vi "PathfinderUtil_ToTrajectoryStates.vi"(11 "Pathfinder Path":T1[](array[typedef])) -> (3 "TrajectoryStates":T2[](array[typedef]) {"POSE"."ROTATION"."SIN" format="%13.4f"; "POSE"."ROTATION"."COS" format="%13.4f"; "POSE"."ROTATION"."VALUE" format="%13.4f"; "POSE"."TRANSLATION"."Y" format="%14.3f"; "POSE"."TRANSLATION"."X" format="%14.3f"})   [LabVIEW 2019, in "Trajectory_Library.lvlib"]
doc: "Convert an array of Pathfinder created Path states to an array of Trajectory States. Inches are converted to Meters. Angles are converted to headings (+/- PI). This routine only does a portion of the work needed to convert a Pathfinder Path to a complete Trajectory. (See PathfinderUtil_ToTrajectory for a complete routine.)\n\nParameters:\n - Pathfinder Path - Array of pathfinder created states\n\nReturns:\n - Trajectory States - Array of Trajectory states."
uses:
  Trajectory_Library.lvlib
  TRAJ_STATE.ctl
  POSE2D.ctl
  TRANSLATION2D.ctl
  ROTATION2D.ctl
  Pathfinder-Lib/VIs/Segment.ctl
  Rotation_CreateAngle.vi
  Translation_Create.vi
  Pathfinder-Lib/Pathfinder.lvlib
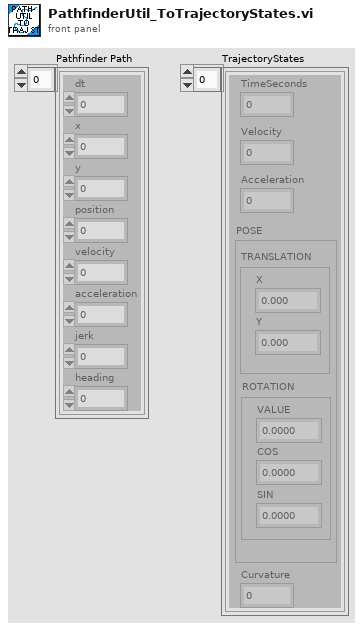
[diagram p1: front panel]
types:
  T1 = typedef "Pathfinder.lvlib/Segment.ctl" = cluster{"dt":dbl, "x":dbl, "y":dbl, "position":dbl, "velocity":dbl, "acceleration":dbl, "jerk":dbl, "heading":dbl}
  T2 = typedef "Trajectory_Library.lvlib/TRAJ_STATE.ctl" = cluster{"TimeSeconds":dbl, "Velocity":dbl, "Acceleration":dbl, "POSE":T3, "Curvature":dbl}
  T3 = typedef "Trajectory_Library.lvlib/POSE2D.ctl" = cluster{"TRANSLATION":T4, "ROTATION":T5}
  T4 = typedef "Trajectory_Library.lvlib/TRANSLATION2D.ctl" = cluster{"X":dbl, "Y":dbl}
  T5 = typedef "Trajectory_Library.lvlib/ROTATION2D.ctl" = cluster{"VALUE":dbl, "COS":dbl, "SIN":dbl}
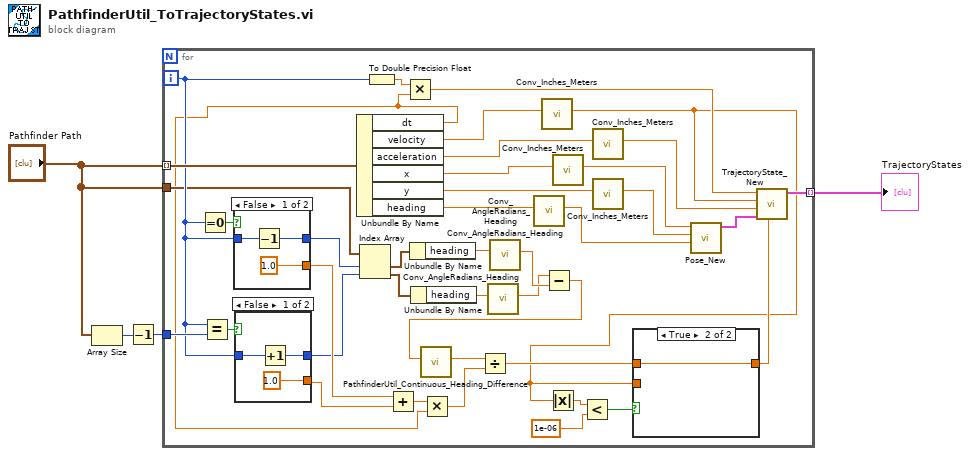
[diagram p0: block diagram]
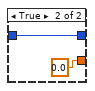
[diagram p2: hidden frame]
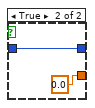
[diagram p3: hidden frame]
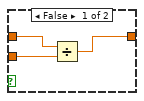
[diagram p4: hidden frame]
diagram:
  n1 = Array Size(array="Pathfinder Path") -> (size(s)=w2:i32)
  n2 = Decrement(x=w2) -> (x-1=w3:i32)
  n3 = for {
    tunnel: "Pathfinder Path" -> [w43] mode=indexing
    tunnel: [w42] -> w4 mode=indexing
    tunnel: "Pathfinder Path" -> [w18]
    tunnel: w3 -> [w26]
    i -> [w25]
    n4 = Equal To 0?(x=w25) -> (x = 0?=w28:bool)
    n5 = Equal?(x=w25, y=w26) -> (x = y?=w27:bool)
    n6 = case shown="False" w28 {
      tunnel: w25 -> [w52 w53]
      tunnel: [1.0 0.0] -> w21
      tunnel: [w50 w53] -> w20
      frame False {
        n7 = Decrement(x=w52) -> (x-1=w50:i32)
      }
      frame True {
      }
    }
    n8 = case shown="False" w27 {
      tunnel: [1.0 0.0] -> w22
      tunnel: w25 -> [w46 w48]
      tunnel: [w45 w48] -> w19
      frame False {
        n9 = Increment(x=w46) -> (x+1=w45:i32)
      }
      frame True {
      }
    }
    n10 = Unbundle By Name(w43) -> ("dt"=w5:dbl, "velocity"=w31:dbl, "acceleration"=w33:dbl, "x"=w37:dbl, "y"=w38:dbl, "heading"=w23:dbl)
    n11 = Index Array(array=w18, index #1=w20, index #2=w19) -> (element #1=w17:T1, element #2=w16:T1)
    n12 = To Double Precision Float(number=w25) -> (double precision float=w44:dbl)
    n13 = Add(x=w21, y=w22) -> (x+y=w14:dbl)
    n14 = Multiply(x=w44, y=w5) -> (x*y=w40:dbl)
    n15 = Unbundle By Name(w17) -> ("heading"=w10:dbl)
    n16 = Unbundle By Name(w16) -> ("heading"=w9:dbl)
    n17 = Multiply(x=w14, y=w5) -> (x*y=w24:dbl)
    n18 = call "Conv_AngleRadians_Heading.vi"("Radians"=w9) -> ("Heading"=w6:dbl)  [unwired: 10 in]
    n19 = call "Conv_AngleRadians_Heading.vi"("Radians"=w10) -> ("Heading"=w7:dbl)  [unwired: 10 in]
    n20 = call "Conv_AngleRadians_Heading.vi"("Radians"=w23) -> ("Heading"=w30:dbl)  [unwired: 10 in]
    n21 = call "Conv_Inches_Meters.vi"("INCH"=w31) -> ("Meters"=w8:dbl)  [unwired: 10 in]
    n22 = Subtract(x=w6, y=w7) -> (x-y=w15:dbl)
    n23 = call "PathfinderUtil_Continuous_Heading_Difference.vi"("Heading Diff"=w15) -> ("Heading Diff"=w29:dbl)  [unwired: 10 in]
    n24 = Divide(x=w29, y=w24) -> (x/y=w39:dbl)
    n25 = Absolute Value(x=w8) -> (abs(x)=w13:dbl)
    n26 = call "Conv_Inches_Meters.vi"("INCH"=w37) -> ("Meters"=w34:dbl)  [unwired: 10 in]
    n27 = Less?(x=w13, y=1e-06) -> (x < y?=w11:bool)
    n28 = call "Conv_Inches_Meters.vi"("INCH"=w33) -> ("Meters"=w32:dbl)  [unwired: 10 in]
    n29 = call "Conv_Inches_Meters.vi"("INCH"=w38) -> ("Meters"=w35:dbl)  [unwired: 10 in]
    n30 = case shown="True" w11 {
      tunnel: w39 -> [w57 w58]
      tunnel: [w55 w58] -> w36
      tunnel: w8 -> [w56 _]
      frame False {
        n31 = Divide(x=w57, y=w56) -> (x/y=w55:dbl)
      }
      frame True {
      }
    }
    n32 = call "Pose_New.vi"("Heading"=w30, "Y"=w35, "X"=w34) -> ("out POSe"=w41:T3)  [unwired: 8 in]
    n33 = call "TrajectoryState_New.vi"("Curvature"=w36, "POSE"=w41, "Accel"=w32, "Velocity"=w8, "Time"=w40) -> ("TRAJ_STATE"=w42:T2)  [unwired: 6 in]
  }
  "TrajectoryStates" <- w4
